vi "Transform_Create_PosePose.vi"(9 "last POSE":T1, 11 "initial POSE":T1) -> (3 "TRANSFORM":T4)   [LabVIEW 2019, in "PathExecution_Library.lvlib"]
uses:
  PathExecution_Library.lvlib
  TRANSFORM.ctl
  TRANSLATION.ctl
  ROTATION.ctl
  POSE.ctl
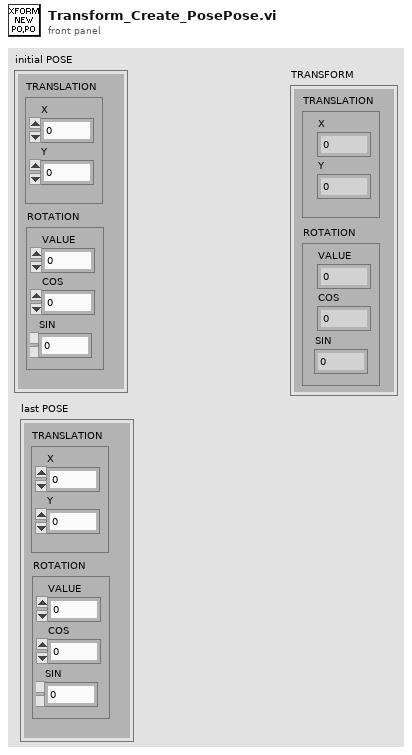
[diagram p1: front panel]
types:
  T1 = typedef "PathExecution_Library.lvlib/POSE.ctl" = cluster{"TRANSLATION":T2, "ROTATION":T3}
  T2 = typedef "PathExecution_Library.lvlib/TRANSLATION.ctl" = cluster{"X":dbl, "Y":dbl}
  T3 = typedef "PathExecution_Library.lvlib/ROTATION.ctl" = cluster{"VALUE":dbl, "COS":dbl, "SIN":dbl}
  T4 = typedef "PathExecution_Library.lvlib/TRANSFORM.ctl" = cluster{"TRANSLATION":T2, "ROTATION":T3}
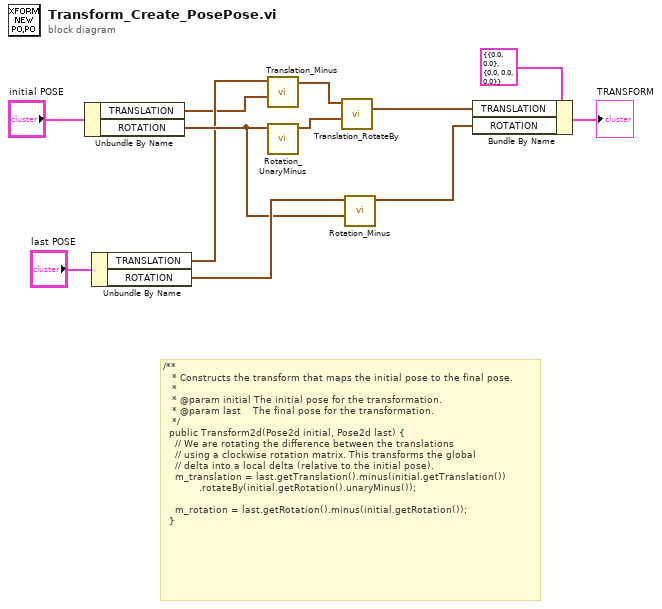
[diagram p0: block diagram]
diagram:
  # "/**\n   * Constructs the transform that maps the initial pose to the final pose.\n   *\n   * @param initial The initial pose for the transformation.\n   * @param last    The final pose for the transformation.\n   */\n  public Transform2d(Pose2d initial, Pose2d last) {\n    // We are rotating the difference between the translations\n    // using a clockwise rotation matrix. This transforms the global\n    // delta into a local delta (relative to the initial pose).\n    m_translation = last.getTranslation().minus(initial.getTranslation())\n            .rotateBy(initial.getRotation().unaryMinus());\n\n    m_rotation = last.getRotation().minus(initial.getRotation());\n  }"
  n1 = Unbundle By Name("initial POSE") -> ("TRANSLATION"=w3:T2, "ROTATION"=w6:T3)
  n2 = Unbundle By Name("last POSE") -> ("TRANSLATION"=w4:T2, "ROTATION"=w7:T3)
  n3 = call "Translation_Minus.vi"("other Translation"=w3, "In Translation"=w4) -> ("Out Translation"=w2:T2)  [unwired: 9 in]
  n4 = call "Rotation_UnaryMinus.vi"("in ROTATION"=w6) -> ("out ROTATION"=w9:T3)  [unwired: 10 in]
  n5 = call "Translation_RotateBy.vi"("other Rotation"=w9, "In Translation"=w2) -> ("Out Translation"=w1:T2)  [unwired: 9 in]
  n6 = call "Rotation_Minus.vi"("other ROTATION"=w6, "in ROTATION"=w7) -> ("out ROTATION"=w5:T3)  [unwired: 9 in]
  n7 = Bundle By Name(cluster=T4 {"TRANSLATION"={"X"=0.0, "Y"=0.0}, "ROTATION"={"VALUE"=0.0, "COS"=0.0, "SIN"=0.0}} ("TRANSFORM"), "TRANSLATION"=w1, "ROTATION"=w5) -> (→"TRANSFORM":T4)
